vi "001 SumaRestaOriol.vi"() -> ()   [LabVIEW 2019]
panel:
  in  "Nombre1":dbl
  in  "Nombre2":dbl
  out "Suma":dbl
  out "Numeric Indicator":dbl
  in  "?":bool
  out "Execucions":i32
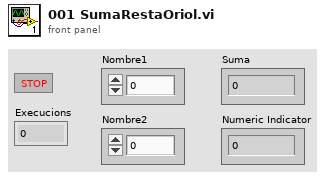
[diagram p1: front panel]
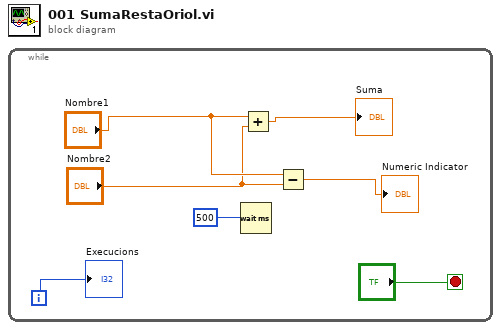
[diagram p0: block diagram]
diagram:
  n1 = while {
    i -> [w1]
    stop <- "?" stop-if-true
    n2 = Wait (ms)(milliseconds to wait=500) -> ()  [unwired: 1 out]
    n3 = Add(x="Nombre1", y="Nombre2") -> (x+y=→"Suma":dbl)
    n4 = Subtract(x="Nombre1", y="Nombre2") -> (x-y=→"Numeric Indicator":dbl)
    "Execucions" <- w1
  }
